vi "Read-Panes.vi"(8 "error in (no error)":errorcluster, 11 "Panes in":refnum<class "SC-UI.lvclass">) -> (0 "error out":errorcluster, 2 "Panes":T1[](array[typedef]), 3 "Panes out":refnum<class "SC-UI.lvclass">)   [LabVIEW 2013, in "SLMControl.lvlib" / "SC-UI.lvclass"]
uses:
  SC-UI.lvclass
  Pane-settings.ctl
  Pane-names.ctl
  Splitter-settings.ctl
  Splitter-names.ctl
  SC-UI.lvclass/SC-UI.ctl
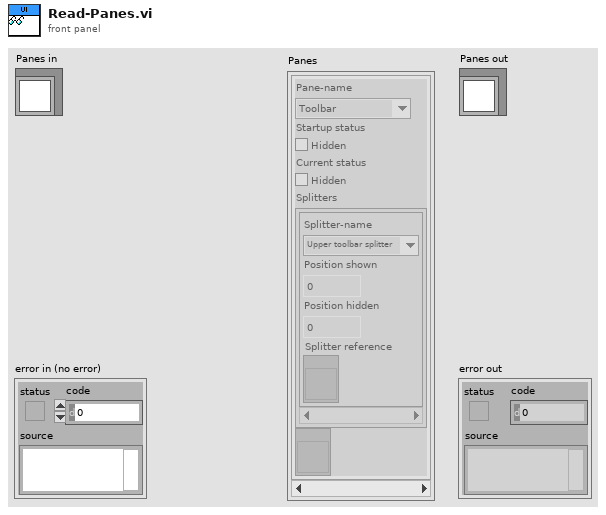
[diagram p1: front panel]
types:
  T1 = typedef "SLMControl.lvlib/SC-UI.lvclass/Pane-settings.ctl" = cluster{"Pane-name":T2, "Startup status":bool, "Current status":bool, "Splitters":T3[], "Pane-reference":refnum<vi>}
  T2 = typedef "SLMControl.lvlib/SC-UI.lvclass/Pane-names.ctl" = enum16{"Toolbar", "Help bar", "Toolbar lower border", "Center panel", "Main panel", "Status panel", "Status bar upper border", "General state bar", "Information bar"}
  T3 = typedef "SLMControl.lvlib/SC-UI.lvclass/Splitter-settings.ctl" = cluster{"Splitter-name":T4, "Position shown":i32, "Position hidden":i32, "Splitter reference":refnum<vi>}
  T4 = typedef "SLMControl.lvlib/SC-UI.lvclass/Splitter-names.ctl" = enum16{"Upper toolbar splitter", "Help bar splitter", "Lower toolbar splitter", "Upper status bar splitter", "Lower status bar splitter", "Left status bar splitter", "Status splitter"}
  T5 = typedef "SLMControl.lvlib/BC-UI.lvclass/Pane-settings.ctl" = cluster{"Pane-name":T6, "Startup status":bool, "Current status":bool, "Splitters":T7[], "Pane-reference":refnum<vi>}
  T6 = typedef "SLMControl.lvlib/BC-UI.lvclass/Pane-names.ctl" = enum16{"Toolbar", "Help bar", "Toolbar lower border", "Center panel", "Main panel", "Status panel", "Status bar upper border", "General state bar", "Information bar"}
  T7 = typedef "SLMControl.lvlib/BC-UI.lvclass/Splitter-settings.ctl" = cluster{"Splitter-name":T8, "Position shown":i32, "Position hidden":i32, "Splitter reference":refnum<vi>}
  T8 = typedef "SLMControl.lvlib/BC-UI.lvclass/Splitter-names.ctl" = enum16{"Upper toolbar splitter", "Help bar splitter", "Lower toolbar splitter", "Upper status bar splitter", "Lower status bar splitter", "Left status bar splitter", "Status splitter"}
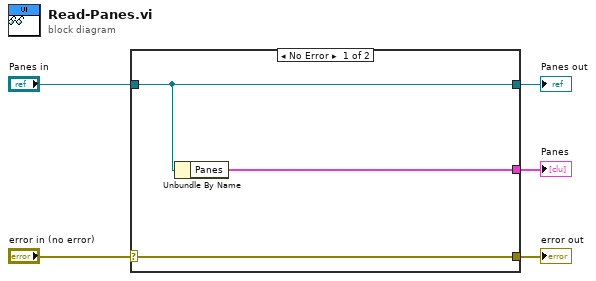
[diagram p0: block diagram]
diagram:
  n1 = case shown="No Error" "error in (no error)" {
    selector: "error in (no error)" -> [w8 w9]
    tunnel: [w8 w9] -> w4
    tunnel: [w7 w10] -> w2
    tunnel: "Panes in" -> [w7 w10]
    tunnel: [w6 _] -> w1
    frame No Error {
      n2 = Unbundle By Name(w7) -> ("Panes"=w6:T5[])
    }
    frame Error {
    }
  }
  "error out" <- w4
  "Panes out" <- w2
  "Panes" <- w1
